vi "Sys-Error Query.vi"(8 "error in (no error)":errorcluster, 9 "source (Sys-Error Query.vi)":string="Sys-Error Query.vi", 11 "VISA session":refnum<visa-resource-name>) -> (0 "error out":errorcluster, 1 "messages":string, 3 "VISA resource name out":refnum<visa-resource-name>)   [LabVIEW 2016, in "Agilent 415X Series.lvlib"]
doc: "This VI reads the status message from the power meter and determines whether an error has occurred during the previous operations. If an error is detected, the messages will be displayed."
uses:
  Agilent 415X Series.lvlib
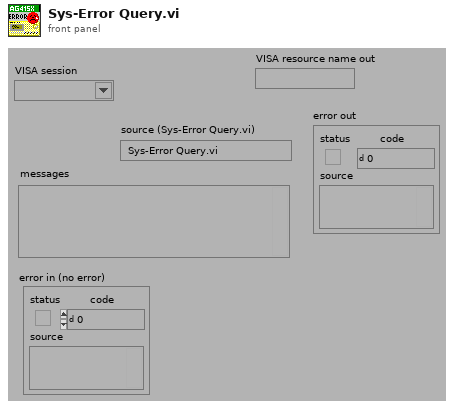
[diagram p1: front panel]
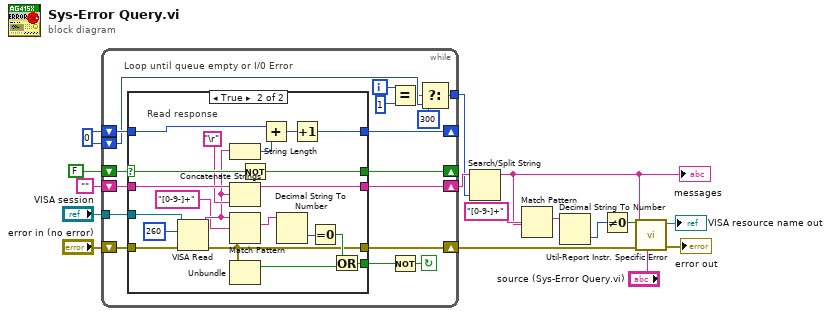
[diagram p0: block diagram]
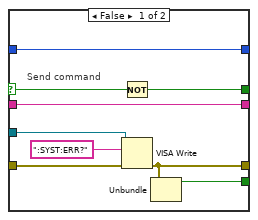
[diagram p2: hidden frame]
diagram:
  w14 = 0
  n1 = while {
    tunnel: "VISA session" -> [w17]
    tunnel: [w22] -> w12
    shift-left: w14 -> [w23]
    shift-left: w14 -> [w25]
    shift-right: [w24] -> _
    shift-left: "error in (no error)" -> [w27]
    shift-right: [w26] -> w5
    shift-left: FALSE -> [w29]
    shift-right: [w28] -> _
    shift-left: "" -> [w32]
    shift-right: [w33] -> w13
    i -> [w21]
    stop <- w30 continue-if-true
    # "Loop until queue empty or I/0 Error"
    n2 = case shown="True" w29 {
      selector: w29 -> [w41 w58]
      tunnel: [w38 w61] -> w31
      tunnel: [w42 w60] -> w33
      tunnel: w32 -> [w42 w59]
      tunnel: [w40 w57] -> w28
      tunnel: [w36 w54] -> w26
      tunnel: w27 -> [w37 w52]
      tunnel: w25 -> [w35 w50]
      tunnel: [w35 w48] -> w24
      tunnel: w17 -> [w34 w43]
      frame False {
        # "Send command"
        n3 = Not(x=w41) -> (.not. x?=w40:bool)
        n4 = VISA Write(VISA resource name=w34, write buffer=":SYST:ERR?", error in (no error)=w37) -> (error out=w36:errorcluster)  [unwired: 2 out]
        n5 = Unbundle(w36) -> ("status"=w38:bool)  [unwired: 2 out]
      }
      frame True {
        # "Read response"
        n6 = VISA Read(VISA resource name=w43, byte count=260, error in (no error)=w52) -> (read buffer=w47:string, error out=w54:errorcluster)  [unwired: 2 out]
        n7 = String Length(string=w47) -> (length=w51:i32)
        n8 = Concatenate Strings(w59, w47, "\r") -> (w60:string)
        n9 = Match Pattern(string=w47, regular expression="[0-9-]+") -> (match substring=w45:string)  [unwired: 1 in, 3 out]
        n10 = Unbundle(w54) -> ("status"=w53:bool)  [unwired: 2 out]
        n11 = Not(x=w58) -> (.not. x?=w57:bool)
        n12 = Add(x=w50, y=w51) -> (x+y=w49:i32)
        n13 = Decimal String To Number(string=w45) -> (number=w62:i32)  [unwired: 2 in, 1 out]
        n14 = Increment(x=w49) -> (x+1=w48:i32)
        n15 = Equal To 0?(x=w62) -> (x = 0?=w56:bool)
        n16 = Or(x=w56, y=w53) -> (x .or. y?=w61:bool)
      }
    }
    n17 = Equal?(x=w21, y=1) -> (x = y?=w19:bool)
    n18 = Not(x=w31) -> (.not. x?=w30:bool)
    n19 = Select(t=300, s=w19, f=w23) -> (s? t:f=w22:i32)
  }
  n20 = Search/Split String(string=w13, offset (0)=w12) -> (substring before match=w3:string)  [unwired: 1 in, 2 out]
  "messages" <- w3
  n21 = Match Pattern(string=w3, regular expression="[0-9-]+") -> (match substring=w10:string)  [unwired: 1 in, 3 out]
  n22 = Decimal String To Number(string=w10) -> (number=w8:i32)  [unwired: 2 in, 1 out]
  n23 = Not Equal To 0?(x=w8) -> (x != 0?=w7:bool)
  n24 = call "Util-Report Instr. Specific Error.vi"("source"="source (Sys-Error Query.vi)", "error in (no error)"=w5, "error message"=w3, "new error"=w7) -> ("error out"=→"error out":errorcluster, "VISA resource name out"=→"VISA resource name out":refnum<visa-resource-name>)  [unwired: 6 in]
